vi "Get Clicked Index.vi"(1 "Element Height (48px)":i32=48, 2 "Refnum in":refnum<vi>) -> (0 "Index":u32)   [LabVIEW 2019, in "UI.lvlib"]
uses:
  UI.lvlib
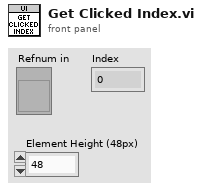
[diagram p1: front panel]
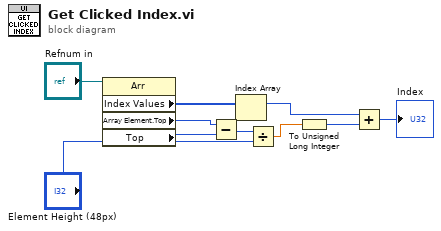
[diagram p0: block diagram]
diagram:
  n1 = property on="Property Node" class="Arr"(reference="Refnum in") -> ("Index Values"=w7:u32[], "Array Element.Top"=w2:i32, "Top"=w3:i32)  [unwired: 1 in, 2 out]
  n2 = Subtract(x=w2, y=w3) -> (x-y=w4:i32)
  n3 = Index Array(array=w7) -> (element=w8:u32)  [unwired: 1 in]
  n4 = Divide(x=w4, y="Element Height (48px)") -> (x/y=w6:dbl)
  n5 = To Unsigned Long Integer(number=w6) -> (unsigned 32bit integer=w9:u32)
  n6 = Add(x=w8, y=w9) -> (x+y=→"Index":u32)
